vi "Release.vi"(8 "Error Input":errorcluster, 10 "Queue In":refnum<queue>, 11 "LiteAgentSDK Input":refnum<k24>) -> (0 "Error Output":errorcluster)   [LabVIEW 2017, in "LiteAgentSDK.lvlib"]
uses:
  LiteAgentSDK.lvlib
  C:/Users/Jan/Projects/LiteAgentSDK-LabVIEW/Source/Bin/LiteAgentSDK.LabVIEW.dll
  Bin/LiteAgentSDK.LabVIEW.dll
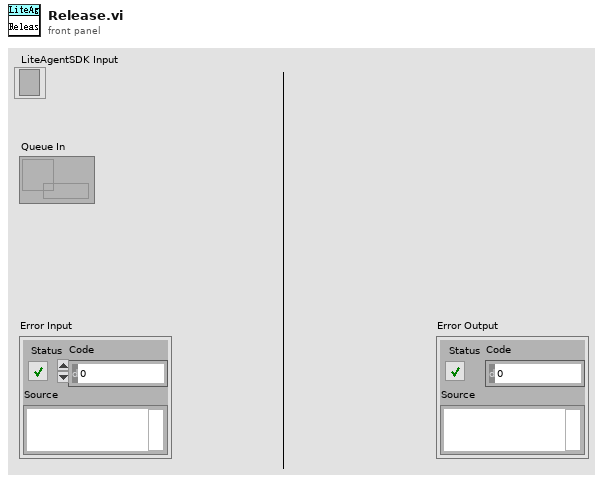
[diagram p1: front panel]
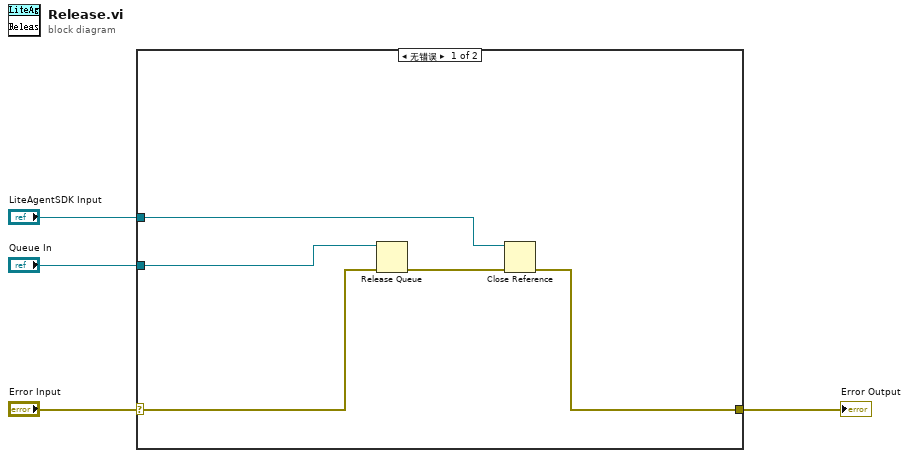
[diagram p0: block diagram]
diagram:
  n1 = case shown="无错误" "Error Input" {
    selector: "Error Input" -> [w8 w10]
    tunnel: [w5 w10] -> w3
    tunnel: "LiteAgentSDK Input" -> [w6 _]
    tunnel: "Queue In" -> [w9 _]
    frame No Error {
      n2 = Release Queue(queue=w9, error in (no error)=w8) -> (error out=w7:errorcluster)  [unwired: 1 in, 2 out]
      n3 = Close Reference(reference=w6, error in (no error)=w7) -> (error out=w5:errorcluster)
    }
    frame Error {
    }
  }
  "Error Output" <- w3
